vi "niScope EX Configured Acquisition_V2.vi"() -> ()   [LabVIEW 2024]
doc: "Recommended Input Signal: 100 kHz, 4 Vpp, sine wave\n\nDevices Supported: Refer to NI Example Finder\n\nThis example configures all the oscilloscope's vertical, horizontal, and triggering properties before every acquisition. It allows you to experiment with numerous configurations, including acquisition types and triggering modes, since it supports nearly the entire functionality of NI-SCOPE. However, it is may be more instructive to consult other examples about specific topics such as FlexRes, Random Interleaved Sampling, and Multi-Record to learn more about these features.\n\nMany parameters are included an the front panel of this example. Notice that the \"min sample rate\" is next to the \"actual sample rate,\" and similarly the \"min record length\" is near the \"actual record length.\" The \"min\" values are specified with the Configure Horizontal Timing VI. NI-SCOPE maintains a constant time per record for each acquisition. So when you specify a min sample rate and a min record length, this determines the amount of time the acquisition should take:\n\n time per record = min record length / min sampling rate. \n\nHowever, oscilloscopes support only a certain number of defined sampling rates, so if the value chosen is not a valid rate, it is rounded to the next higher rate, called the actual sample rate. The actual record length is then calculated in order to maintain the time per record. Both of these values are returned in this example so you can investigate the effects of parameter rounding with your oscilloscope. For more information about parameter coercions, see the NI High Speed Digitizers Help.\n\nThe enforce realtime property allows this example to use Random Interleaved Sampling. See the Random Interleaved Sampling example for more details.\n\nKeep in mind that not all digitizers/oscilloscopes support all the features in this example. The NI High Speed Digitizers Help includes a table of supported features for each device."
uses:
  <instrlib>/niScope/Utility/niScope Get Channel Name From String.vi
  <instrlib>/niScope/Configure/Trigger/niScope Configure Trigger Immediate.vi
  <instrlib>/niScope/Configure/Trigger/niScope Configure Trigger Edge.vi
  <instrlib>/niScope/Configure/Trigger/niScope Configure Trigger Digital.vi
  <instrlib>/niScope/Configure/Trigger/niScope Configure Trigger Window.vi
  <instrlib>/niScope/Configure/Trigger/niScope Configure Trigger Hysteresis.vi
  <instrlib>/niScope/Acquire/Fetch/niScope Multi Fetch WDT.vi
panel:
  out "Waveform Graph":waveform(dbl)[](graph)
  in  "Trigger Type":T1(tab)
  in  "Trigger Source":string(combo)="0"
  in  "Trigger Level":dbl format="%.2f"
  in  "Trigger Slope":i32(ring) items=["Positive", "Negative"]
  in  "Coupling":u16(ring)=1 caption="Trigger Coupling" items=["AC"=0, "DC"=1, "HF Reject"=3, "LF Reject"=4, "AC Plus HF Reject"=1001]
  in  "Trigger Slope":i32(ring) items=["Positive", "Negative"]
  in  "Trigger Source":string(combo)="VAL_PFI_1"
  in  "Coupling":u16(ring)=1 caption="Trigger Coupling" items=["AC"=0, "DC"=1, "HF Reject"=3, "LF Reject"=4, "AC Plus HF Reject"=1001]
  in  "High Level":dbl=0.1 caption="Window High Level" format="%.2f"
  in  "Low Level":dbl=-0.1 caption="Window Low Level" format="%.2f"
  in  "Window Mode":i32(ring) items=["Entering", "Leaving"]
  in  "Trigger Source":string(combo)="0"
  in  "Hysteresis":dbl=0.05 format="%.2f"
  in  "Trigger Source":string(combo)="0"
  in  "Trigger Level":dbl format="%.2f"
  in  "Coupling":u16(ring)=1 caption="Trigger Coupling" items=["AC"=0, "DC"=1, "HF Reject"=3, "LF Reject"=4, "AC Plus HF Reject"=1001]
  in  "Trigger Slope":i32(ring) items=["Positive", "Negative"]
  out "Auto Triggered":bool
  in  "Trigger Modifier":i32(ring)=2 items=["None"=1, "Auto Trigger"=2]
  in  "Vertical Coupling":i32(ring)=1 items=["AC", "DC", "Ground"]
  in  "Stop":bool
  in  "Reference Position":dbl=50.0 caption="Ref Position" format="%.1f"
  in  "Trigger Delay":dbl caption="Trigger Delay (s)" format="%#.4p"
  in  "Maximum Input Frequency":dbl caption="Max. Input Frequency (Hz)" format="%.2f"
  in  "Input Impedance":u32(ring) items=["1 mega ohm"=0, "50 ohms"=2]
  in  "Probe Attenuation":dbl=1.0 format="%.1f"
  in  "Vertical Offset":dbl caption="Vertical Offset (V)" format="%.2p"
  out "Actual Sample Rate":dbl=10000000.0 format="%#.2p"
  out "Actual Record Length":i32=1000
  in  "Min Record Length":i32=1000 caption="Min. Record Length"
  in  "Min Sample Rate":dbl=10000000.0 caption="Min. Sample Rate" step=1000000.0 format="%#.2p"
  in  "Vertical Range":dbl=5.0 caption="Vertical Range (V)" format="%.2f"
  in  "Enforce Realtime":bool=TRUE
  in  "Channel Name":string="0" caption="Channel(s)"
  in  "Resource Name":refnum<k15>="Dev1" caption="Resource Name(s)"
  # "Vertical"
  # "Channel"
  # "Trigger"
  # "Common Trigger Settings"
  # "Horizontal"
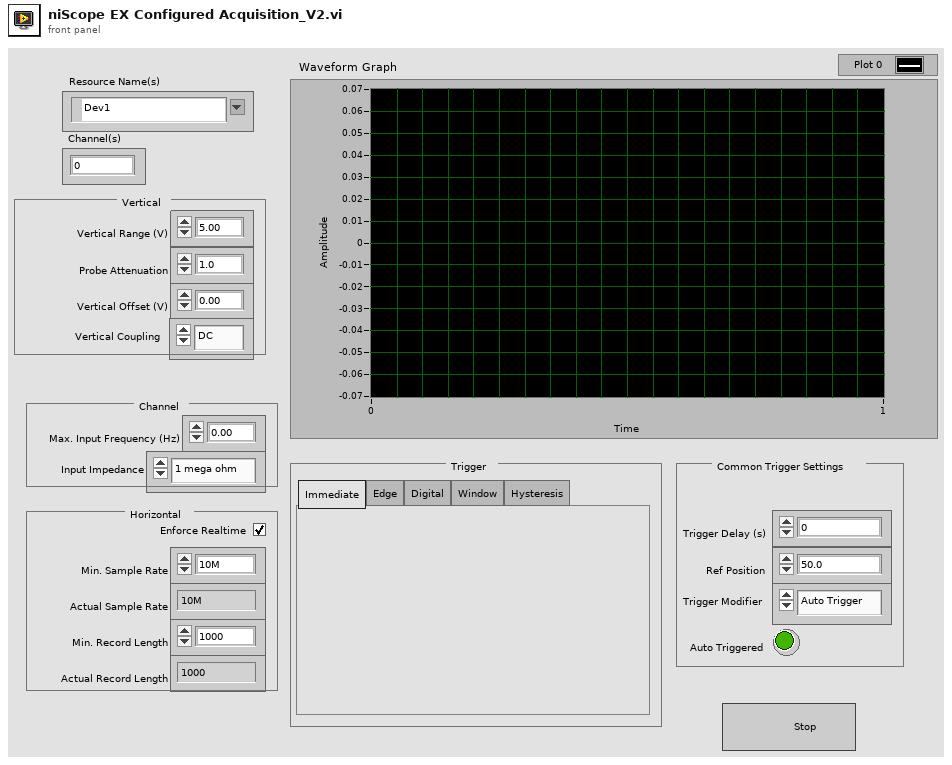
[diagram p1: front panel]
types:
  T1 = enum32{"Immediate", "Edge", "Digital", "Window", "Hysteresis"}
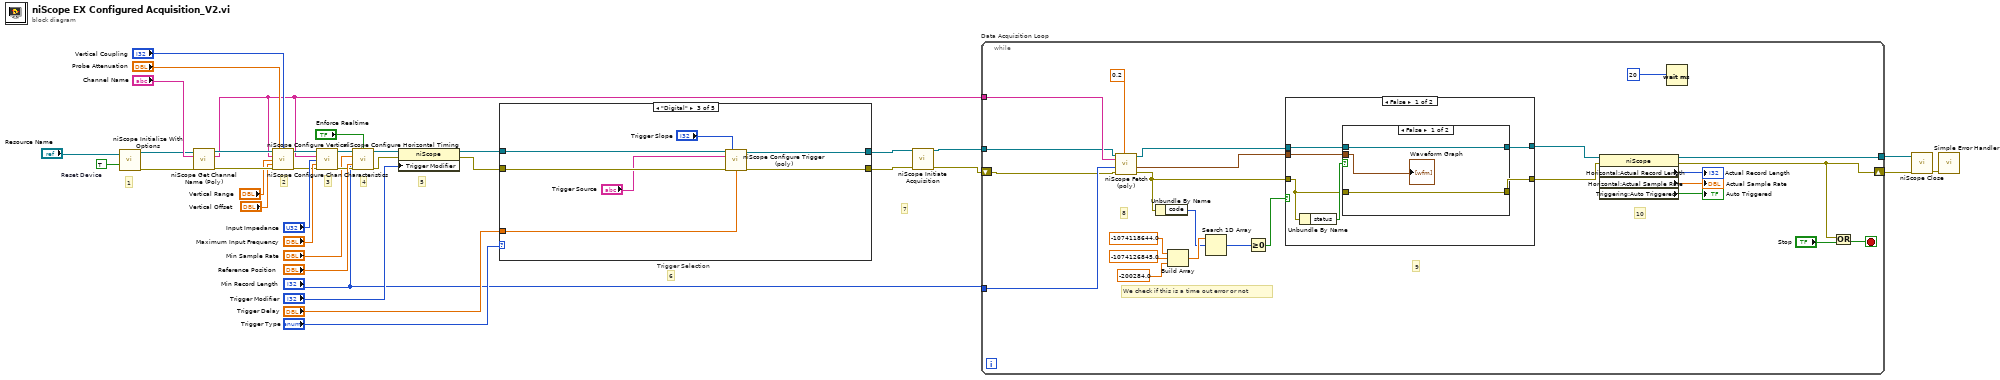
[diagram p0: block diagram]
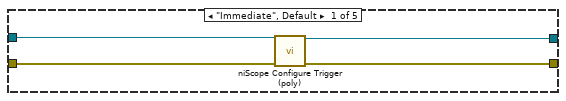
[diagram p2: hidden frame]
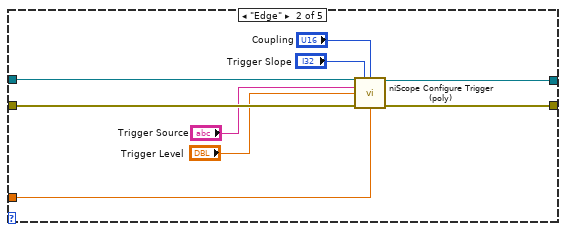
[diagram p3: hidden frame]
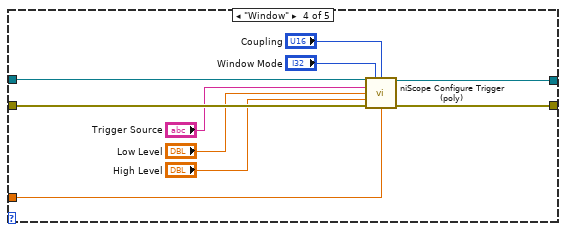
[diagram p4: hidden frame]
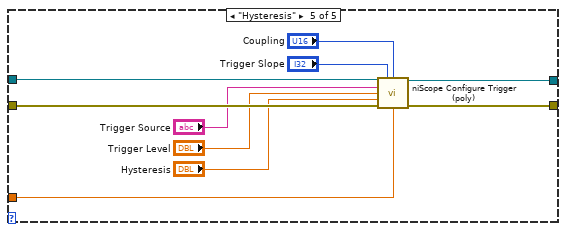
[diagram p5: hidden frame]
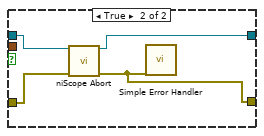
[diagram p6: hidden frame]
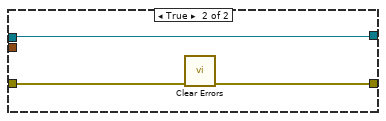
[diagram p7: hidden frame]
diagram:
  w36 = TRUE  # Reset Device
  # "5"
  # "2"
  # "3"
  # "4"
  # "6"
  # "7"
  # "1"
  n1 = call <instrlib>:"niScope Initialize With Options.vi"("resource name"="Resource Name", "reset device"=w36) -> ("instrument handle"=w6:refnum<k15>, "error out"=w5:errorcluster)  [unwired: 12 in]
  n2 = call-poly <instrlib>:"niScope Get Channel Name (Poly).vi"("instrument handle"=w6, "index"="Channel Name", "error in"=w5) -> ("instrument handle out"=w29:refnum<k15>, "channel name"=w4:string, "error out"=w30:errorcluster)  [unwired: 10 in]
  n3 = call <instrlib>:"niScope Configure Vertical.vi"("instrument handle"=w29, "probe attenuation"="Probe Attenuation", "vertical coupling"="Vertical Coupling", "channels"=w4, "vertical range"="Vertical Range", "vertical offset"="Vertical Offset", "error in"=w30) -> ("instrument handle out"=w9:refnum<k15>, "error out"=w10:errorcluster)  [unwired: 7 in]
  n4 = call <instrlib>:"niScope Configure Chan Characteristics.vi"("instrument handle"=w9, "channels"=w4, "input impedance"="Input Impedance", "maximum input frequency"="Maximum Input Frequency", "error in"=w10) -> ("instrument handle out"=w12:refnum<k15>, "error out"=w11:errorcluster)  [unwired: 9 in]
  n5 = call <instrlib>:"niScope Configure Horizontal Timing.vi"("instrument handle"=w12, "enforce realtime"="Enforce Realtime", "min sample rate"="Min Sample Rate", "reference position"="Reference Position", "error in"=w11, "min record length"="Min Record Length") -> ("instrument handle out"=w22:refnum<k15>, "error out"=w23:errorcluster)  [unwired: 8 in]
  n6 = property on="Property Node" class="niScope"(reference=w22, error in=w23, "Trigger Modifier"="Trigger Modifier") -> (reference out=w25:refnum<k15>, error out=w24:errorcluster)
  n7 = case "Trigger Selection" shown="\"Digital\"" "Trigger Type" {
    tunnel: w24 -> [w40 w49 w56 w66 w76]
    tunnel: [w37 w45 w52 w62 w72] -> w20
    tunnel: w25 -> [w39 w48 w55 w65 w75]
    tunnel: [w38 w46 w53 w63 w74] -> w19
    tunnel: "Trigger Delay" -> [_ w47 w54 w64 w73]
    frame "Immediate", Default {
      n8 = call-poly <instrlib>:"niScope Configure Trigger (poly).vi"("instrument handle"=w39, "error in"=w40) -> ("instrument handle out"=w38:refnum<k15>, "error out"=w37:errorcluster)  [unwired: 12 in]
    }
    frame "Edge" {
      n9 = call-poly <instrlib>:"niScope Configure Trigger (poly).vi"("instrument handle"=w48, "trigger slope"="Trigger Slope", "trigger coupling"="Coupling", "trigger source"="Trigger Source", "trigger level"="Trigger Level", "error in"=w49, "trigger delay"=w47) -> ("instrument handle out"=w46:refnum<k15>, "error out"=w45:errorcluster)  [unwired: 7 in]
    }
    frame "Digital" {
      n10 = call-poly <instrlib>:"niScope Configure Trigger (poly).vi"("instrument handle"=w55, "trigger slope"="Trigger Slope", "trigger source"="Trigger Source", "error in"=w56, "trigger delay"=w54) -> ("instrument handle out"=w53:refnum<k15>, "error out"=w52:errorcluster)  [unwired: 9 in]
    }
    frame "Window" {
      n11 = call-poly <instrlib>:"niScope Configure Trigger (poly).vi"("instrument handle"=w65, "trigger window mode"="Window Mode", "trigger coupling"="Coupling", "trigger source"="Trigger Source", "low level"="Low Level", "high level"="High Level", "error in"=w66, "trigger delay"=w64) -> ("instrument handle out"=w63:refnum<k15>, "error out"=w62:errorcluster)  [unwired: 6 in]
    }
    frame "Hysteresis" {
      n12 = call-poly <instrlib>:"niScope Configure Trigger (poly).vi"("instrument handle"=w75, "trigger slope"="Trigger Slope", "trigger coupling"="Coupling", "trigger source"="Trigger Source", "trigger level"="Trigger Level", "hysteresis"="Hysteresis", "error in"=w76, "trigger delay"=w73) -> ("instrument handle out"=w74:refnum<k15>, "error out"=w72:errorcluster)  [unwired: 6 in]
    }
  }
  n13 = call <instrlib>:"niScope Initiate Acquisition.vi"("instrument handle"=w19, "error in"=w20) -> ("instrument handle out"=w3:refnum<k15>, "error out"=w1:errorcluster)  [unwired: 12 in]
  n14 = while "Data Acquisition Loop" {
    tunnel: [w101] -> w34
    shift-right: [w95] -> w33
    shift-left: w1 -> [w77]
    tunnel: w4 -> [w80]
    tunnel: w3 -> [w79]
    tunnel: "Min Record Length" -> [w78]
    stop <- w96 stop-if-true
    # "9"
    # "We check if this is a time out error or not"
    # "8"
    # "10"
    n15 = call-poly <instrlib>:"niScope Fetch (poly).vi"("timeout"=0.2, "error in"=w77, "numSamples"=w78, "channels"=w80, "instrument handle"=w79) -> ("error out"=w87:errorcluster, "wfm"=w83:waveform(dbl)[], "instrument handle out"=w85:refnum<k15>)  [unwired: 3 in, 1 out]
    n16 = Unbundle By Name(w87) -> ("code"=w81:i32)
    n17 = Build Array(-1074118644.0 ("element"), -1074126845.0 ("element"), -200284.0 ("element")) -> (w90:dbl[])
    n18 = Search 1D Array(1D array=w90, element=w81) -> (index of element=w89:i32)  [unwired: 1 in]
    n19 = Greater Or Equal To 0?(x=w89) -> (x >= 0?=w88:bool)
    n20 = case shown="False" w88 {
      tunnel: w87 -> [w103 w117]
      tunnel: [w106 w116] -> w86
      tunnel: w85 -> [w105 w116]
      tunnel: [w104 w115] -> w84
      tunnel: w83 -> [w102 _]
      frame False {
        n21 = Unbundle By Name(w103) -> ("status"=w107:bool)
        n22 = case shown="False" w107 {
          tunnel: [w109 w113] -> w106
          tunnel: w105 -> [w109 w114]
          tunnel: [w108 w111] -> w104
          tunnel: w103 -> [w108 w112]
          tunnel: w102 -> [w110 _]
          frame False {
            "Waveform Graph" <- w110
          }
          frame True {
            n23 = call <instrlib>:"niScope Abort.vi"("instrument handle"=w114, "error in"=w112) -> ("instrument handle out"=w113:refnum<k15>, "error out"=w111:errorcluster)  [unwired: 12 in]
            n24 = call <vilib>:"Simple Error Handler.vi"("error in (no error)"=w111) -> ()  [unwired: 4 in, 5 out]
          }
        }
      }
      frame True {
        n25 = call <vilib>:"Clear Errors.vi"("error in (no error)"=w117) -> ("error out"=w115:errorcluster)  [unwired: 5 in, 1 out]
      }
    }
    n26 = property class="niScope"(reference=w86, error in=w84) -> (reference out=w101:refnum<k15>, error out=w95:errorcluster, "Horizontal:Actual Record Length"=→"Actual Record Length":i32, "Horizontal:Actual Sample Rate"=→"Actual Sample Rate":dbl, "Triggering:Auto Triggered"=→"Auto Triggered":bool)
    n27 = Wait (ms)(milliseconds to wait=u32 20) -> ()  [unwired: 1 out]
    n28 = Or(x=w95, y="Stop") -> (x .or. y?=w96:bool)
  }
  n29 = call <instrlib>:"niScope Close.vi"("instrument handle"=w34, "error in"=w33) -> ("error out"=w35:errorcluster)  [unwired: 13 in]
  n30 = call <vilib>:"Simple Error Handler.vi"("error in (no error)"=w35) -> ()  [unwired: 4 in, 5 out]
